vi "MessageName.vi"(11 "Msg in":refnum<class "Msg.lvclass">) -> (2 "MessageName":string)   [LabVIEW 2023, in "ConstellationCommand.lvlib" / "Msg.lvclass"]
uses:
  Msg.lvclass
  Msg.lvclass/Msg.ctl
  ConstellationCommand.lvlib
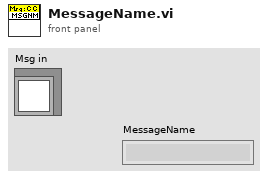
[diagram p1: front panel]
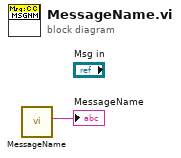
[diagram p0: block diagram]
diagram:
  n1 = call "MessageName.vi"() -> ("MessageName"=→"MessageName":string)  [unwired: 11 in]
